vi "NumberReadMicro.vi"(8 "error in (no error)":errorcluster, 11 "Simulado in":refnum<class "Simulado.lvclass">) -> (0 "error out":errorcluster, 2 "Number":string, 3 "Simulado out":refnum<class "Simulado.lvclass">)   [LabVIEW 2020, in "Simulado.lvclass"]
uses:
  Simulado.lvclass
  Abstract/Serial Device/Serial Device.lvclass
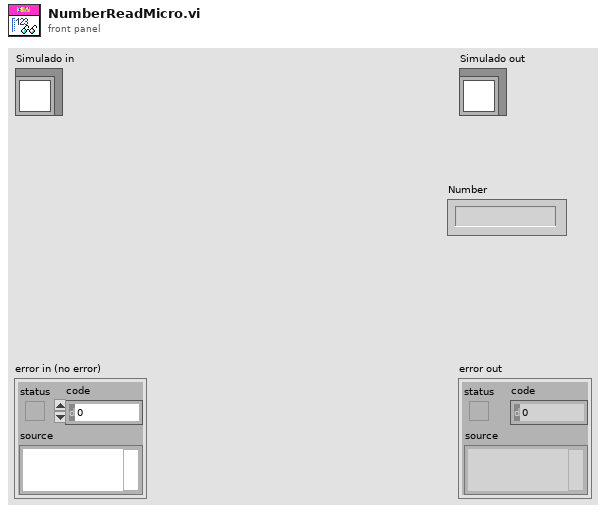
[diagram p1: front panel]
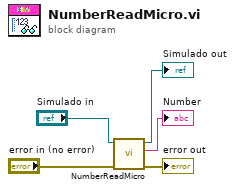
[diagram p0: block diagram]
diagram:
  n1 = call-parent "NumberReadMicro.vi"("error in (no error)"="error in (no error)", "Serial Device in"="Simulado in") -> ("error out"=→"error out":errorcluster, "Number"=→"Number":string, "Serial Device out"=→"Simulado out":refnum<class "Simulado.lvclass">)  [unwired: 7 in]
